vi "Thorlabs_CCS_Connect.vi"(0 "USB VISA Resource Name":string, 1 "Top VI reference":refnum<vi>, 7 "Auto detect USB devices":bool, 11 "error in (no error)":errorcluster) -> (4 "Instrument Refnum":refnum<visa-resource-name>, 6 "Detector":T1, 15 "error out":errorcluster)   [LabVIEW 2021]
doc: "Connects to the instrument via USB and returns the instrument refnum and the detector infos.\n\nIf the \"Auto detect USB devices\" input is false, you must provide a valid \"USB VISA Resource Name\".\n\nIf the \"Auto detect USB devices\" input is true, you must provide a VI reference of the top VI at the \"Top VI reference\" input. The VI reference is used to create a busy cursor when searching for instruments."
uses:
  _Controls/Thorlabs_CCS_Detector_Info.ctl
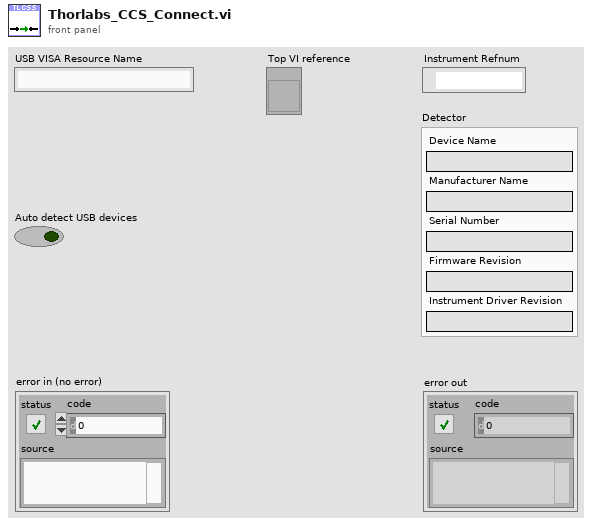
[diagram p1: front panel]
types:
  T1 = typedef "Thorlabs_CCS_Detector_Info.ctl" = cluster{"Device Name":string, "Manufacturer Name":string, "Serial Number":string, "Firmware Revision":string, "Instrument Driver Revision":string}
  T2 = cluster{"Device Name":string, "Manufacturer Name":string, "Serial Number":string, "Firmware Revision":string, "Instrument Driver Revision":string}
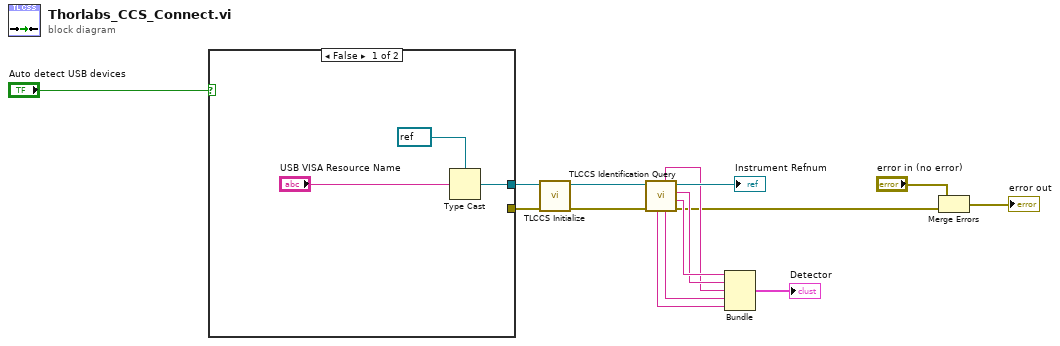
[diagram p0: block diagram]
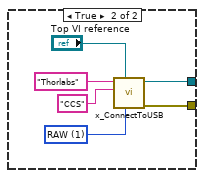
[diagram p2: hidden frame]
diagram:
  n1 = case shown="False" "Auto detect USB devices" {
    tunnel: [_ w24] -> w12
    tunnel: [w16 w23] -> w11
    frame False {
      n2 = Type Cast(type=refnum<visa-resource-name> refnum ("resource name"), x="USB VISA Resource Name") -> (*(type *) &x=w16:refnum<visa-resource-name>)
    }
    frame True {
      w22 = u16 1 items=["INSTR", "RAW"] ("Instrument Class")
      n3 = call <instrlib>:"x_ConnectToUSB.vi"("Instrument Class"=w22, "VI reference"="Top VI reference", "Model"="CCS", "Manufacturer"="Thorlabs") -> ("error out"=w24:errorcluster, "USB Ref"=w23:refnum<visa-resource-name>)  [unwired: 5 in, 1 out]
    }
  }
  n4 = call <instrlib>:"TLCCS Initialize.vi"("error in (no error)"=w12, "resource name"=w11) -> ("error out"=w14:errorcluster, "instrument handle out"=w13:refnum<visa-resource-name>)  [unwired: 8 in]
  n5 = call <instrlib>:"TLCCS Identification Query.vi"("error in (no error)"=w14, "instrument handle"=w13) -> ("error out"=w4:errorcluster, "Device Name"=w10:string, "Manufacturer Name"=w9:string, "instrument handle out"=→"Instrument Refnum":refnum<visa-resource-name>, "Serial Number"=w8:string, "Firmware Revision"=w7:string, "Instrument Driver Revision"=w6:string)  [unwired: 3 in]
  n6 = Bundle("Device Name"=w10, "Manufacturer Name"=w9, "Serial Number"=w8, "Firmware Revision"=w7, "Instrument Driver Revision"=w6) -> (→"Detector":T2)  [unwired: 1 in]
  n7 = Merge Errors("error in (no error)", w4) -> (→"error out":errorcluster)
